vi "MGI Running Average(DBL[]).vi"(5 "Averaging Size":i32, 6 "Average Type(FIR)":T1, 7 "Initialize? (F)":bool, 11 "Value[i]":dbl[](array[numeric])) -> (3 "Average[i]":dbl[](array[numeric]))   [LabVIEW 2020]
doc: "Keep running averages of each of the input values. Infinite Impulse Response requires less processing, but it takes infinite time to arrive at a steady state value. Finite Impulse Reponse maintains an array of the specified size but is able to output means.\nThis VI is a reentrant functional global.\n\nAuthored by Shawn Walpole\nsupport@mooregoodideas.com\nwww.mooregoodideas.com\n\nCopyright (c) 2010, Moore Good Ideas, Inc.\n\nAll rights reserved.\n\nRedistribution and use in source and binary forms, with or without modification, are permitted provided that the following conditions are met:\n\n * Redistributions of source code must retain the above copyright notice, this list of conditions and the following disclaimer.\n * Redistributions in binary form must reproduce the above copyright notice, this list of conditions and the following disclaimer in the documentation and/or other materials provided with the distribution.\n * Neither the name of Moore Good Ideas, Inc. nor the names of its contributors may be used to endorse or promote products derived from this software without specific prior written permission.\n\nTHIS SOFTWARE IS PROVIDED BY THE COPYRIGHT HOLDERS AND CONTRIBUTORS \"AS IS\" AND ANY EXPRESS OR IMPLIED WARRANTIES, INCLUDING, BUT NOT LIMITED TO, THE IMPLIED WARRANTIES OF MERCHANTABILITY AND FITNESS FOR A PARTICULAR PURPOSE ARE DISCLAIMED. IN NO EVENT SHALL THE COPYRIGHT OWNER OR CONTRIBUTORS BE LIABLE FOR ANY DIRECT, INDIRECT, INCIDENTAL, SPECIAL, EXEMPLARY, OR CONSEQUENTIAL DAMAGES (INCLUDING, BUT NOT LIMITED TO, PROCUREMENT OF SUBSTITUTE GOODS OR SERVICES; LOSS OF USE, DATA, OR PROFITS; OR BUSINESS INTERRUPTION) HOWEVER CAUSED AND ON ANY THEORY OF LIABILITY, WHETHER IN CONTRACT, STRICT LIABILITY, OR TORT (INCLUDING NEGLIGENCE OR OTHERWISE) ARISING IN ANY WAY OUT OF THE USE OF THIS SOFTWARE, EVEN IF ADVISED OF THE POSSIBILITY OF SUCH DAMAGE."
uses:
  <userlib>/_MGI/1D Array/MGI Average Type Enum.ctl
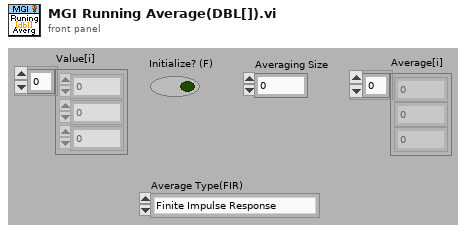
[diagram p1: front panel]
types:
  T1 = typedef "MGI Average Type Enum.ctl" = enum16{"Finite Impulse Response", "Infinite Impulse Response"}
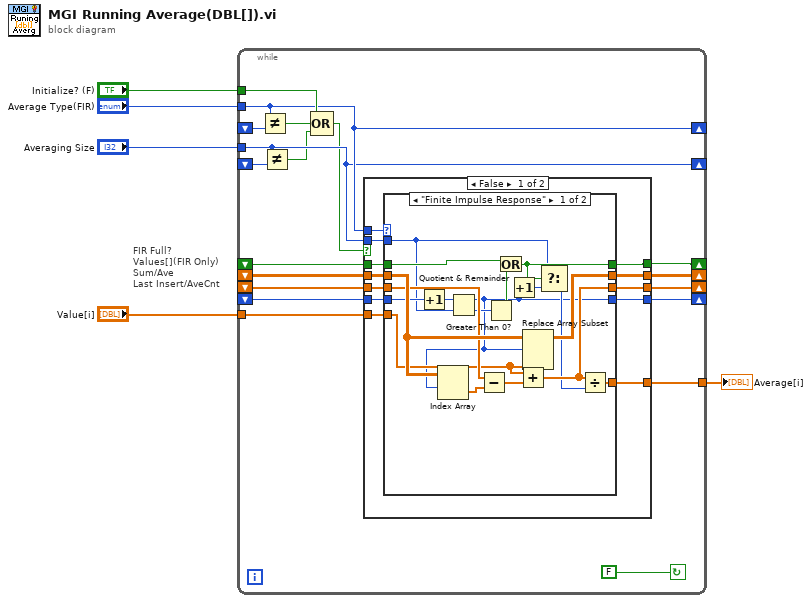
[diagram p0: block diagram]
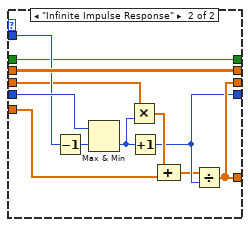
[diagram p2: hidden frame]
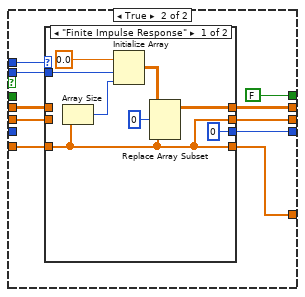
[diagram p3: hidden frame]
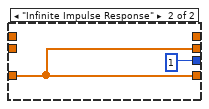
[diagram p4: hidden frame]
diagram:
  # "FIR Full?\nValues[](FIR Only)\nSum/Ave\nLast Insert/AveCnt"
  n1 = while {
    tunnel: "Averaging Size" -> [w13]
    tunnel: "Value[i]" -> [w15]
    shift-left: _ -> [w18]
    shift-right: [w20] -> _
    tunnel: "Initialize? (F)" -> [w22]
    shift-left: _ -> [w9]
    shift-right: [w17] -> _
    tunnel: "Average Type(FIR)" -> [w14]
    shift-right: [w14] -> _
    shift-left: _ -> [w23]
    shift-right: [w21] -> _
    shift-left: _ -> [w19]
    shift-right: [w13] -> _
    shift-left: _ -> [w8]
    tunnel: [w16] -> w3
    shift-right: [w7] -> _
    shift-left: _ -> [w6]
    stop <- FALSE continue-if-true
    n2 = Not Equal?(x=w14, y=w23) -> (x != y?=w12:bool)
    n3 = Not Equal?(x=w13, y=w8) -> (x != y?=w10:bool)
    n4 = Compound Arithmetic op=OR(w22, w12, w10) -> (w11:bool)
    n5 = case shown="False" w11 {
      tunnel: [w30 w68] -> w21
      tunnel: w15 -> [w32 w71]
      tunnel: [w28 w70] -> w20
      tunnel: w19 -> [w35 _]
      tunnel: w18 -> [w34 w74]
      tunnel: w9 -> [w33 w72]
      tunnel: w13 -> [w31 w75]
      tunnel: w14 -> [w36 w76]
      tunnel: [w29 w73] -> w17
      tunnel: [w27 w69] -> w16
      tunnel: [w26 FALSE] -> w7
      tunnel: w6 -> [w25 _]
      frame False {
        n6 = case shown="\"Finite Impulse Response\"" w36 {
          tunnel: w35 -> [w52 w65]
          tunnel: w34 -> [w51 w62]
          tunnel: w33 -> [w53 w66]
          tunnel: w32 -> [w47 w61]
          tunnel: w31 -> [w39 w64]
          tunnel: [w37 w57] -> w30
          tunnel: [w49 w66] -> w29
          tunnel: [w46 w59] -> w28
          tunnel: [w45 w59] -> w27
          tunnel: [w40 w56] -> w26
          tunnel: w25 -> [w41 w56]
          frame "Finite Impulse Response" {
            n7 = Increment(x=w52) -> (x+1=w54:i32)
            n8 = Quotient & Remainder(x=w54, y=w39) -> (x-y*floor(x/y)=w37:i32, floor(x/y)=w42:i32)
            n9 = Index Array(array=w53, index (row)=w37) -> (element=w50:dbl[])  [unwired: 1 in]
            n10 = Subtract(x=w51, y=w50) -> (x-y=w48:dbl[])
            n11 = Greater Than 0?(x=w42) -> (x > 0?=w43:bool)
            n12 = Or(x=w41, y=w43) -> (x .or. y?=w40:bool)
            n13 = Increment(x=w37) -> (x+1=w44:i32)
            n14 = Add(x=w47, y=w48) -> (x+y=w46:dbl[])
            n15 = Replace Array Subset(array=w53, new element=w47, index (row)=w37) -> (w49:dbl[][])  [unwired: 1 in]
            n16 = Select(t=w39, s=w40, f=w44) -> (s? t:f=w38:i32)
            n17 = Divide(x=w46, y=w38) -> (x/y=w45:dbl[])
          }
          frame "Infinite Impulse Response" {
            n18 = Decrement(x=w64) -> (x-1=w63:i32)
            n19 = Max & Min(x=w65, y=w63) -> (min(x,y)=w58:i32)  [unwired: 1 out]
            n20 = Multiply(x=w62, y=w58) -> (x*y=w60:dbl[])
            n21 = Increment(x=w58) -> (x+1=w57:i32)
            n22 = Compound Arithmetic op=ADD(w60, w61) -> (w55:dbl[])
            n23 = Divide(x=w55, y=w57) -> (x/y=w59:dbl[])
          }
        }
      }
      frame True {
        n24 = case shown="\"Finite Impulse Response\"" w76 {
          tunnel: w75 -> [w82 _]
          tunnel: w74 -> [_ _]
          tunnel: [w79 _] -> w73
          tunnel: w72 -> [_ _]
          tunnel: w71 -> [w78 w86]
          tunnel: [w78 w86] -> w70
          tunnel: [w78 w86] -> w69
          tunnel: [0 1] -> w68
          frame "Finite Impulse Response" {
            n25 = Array Size(array=w78) -> (size(s)=w77:i32)
            n26 = Initialize Array(0.0 ("element"), w82, w77) -> (w81:dbl[][])
            n27 = Replace Array Subset(array=w81, new element=w78, index (row)=0 ("index")) -> (w79:dbl[][])  [unwired: 1 in]
          }
          frame "Infinite Impulse Response" {
          }
        }
      }
    }
  }
  "Average[i]" <- w3
